vi "CreatEventsListFireRequestvi.vi"(10 "error in (no error)":errorcluster) -> (2 "error out":errorcluster, 3 "EvnLstFireRqst":T1 caption="EventsListFireRequest")   [LabVIEW 2020, in "CameraTestingProxy.lvlib" / "CameraTestingENI.lvclass"]
uses:
  CameraTestingENI.lvclass
  CameraTestingENI.lvclass/CameraTestingENI.ctl
  Community/TypeDef/RequestEventList.ctl
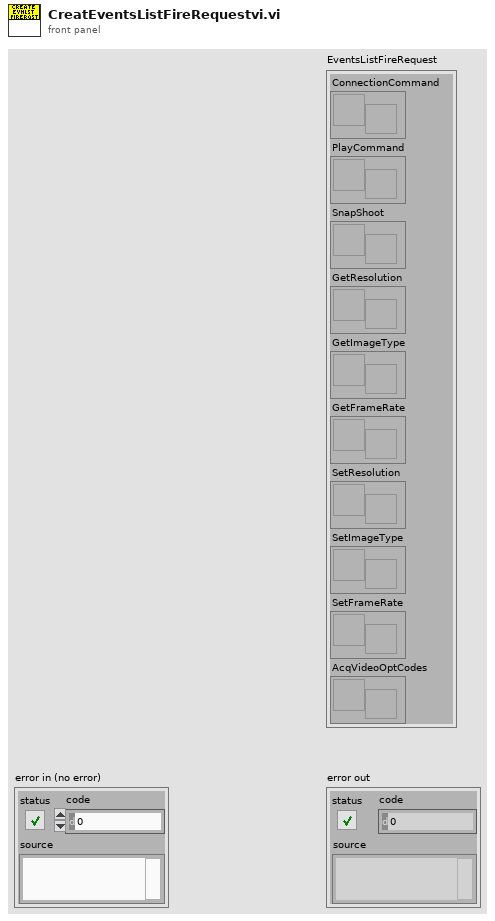
[diagram p1: front panel]
types:
  T1 = typedef "CameraTestingProxy.lvlib/CameraTestingENI.lvclass/RequestEventList.ctl" = cluster{"ConnectCmd":refnum<user-event>, "PlayCmd":refnum<user-event>, "SnapShoot":refnum<user-event>, "GetResolution":refnum<user-event>, "GetImageType":refnum<user-event>, "GetFrameRate":refnum<user-event>, "SetResolution":refnum<user-event>, "SetImageType":refnum<user-event>, "SetFrameRate":refnum<user-event>, "AcqVideoOptCodes":refnum<user-event>}
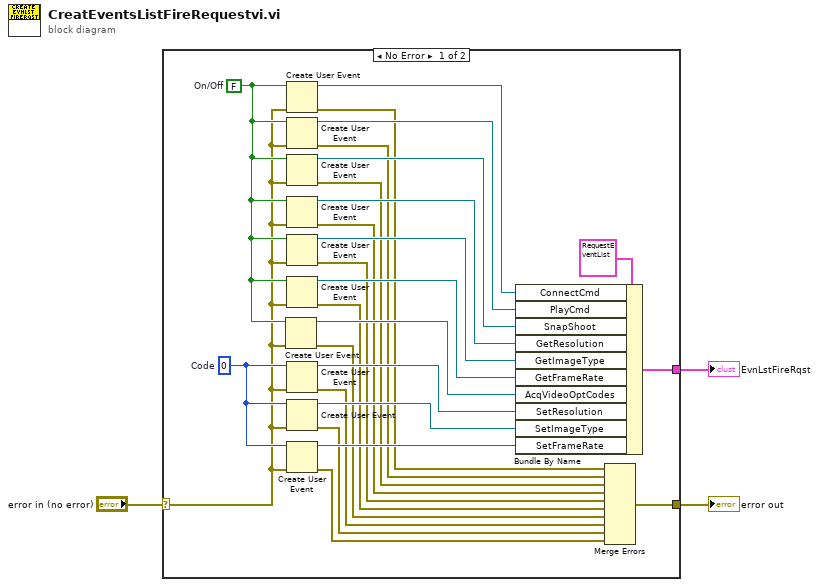
[diagram p0: block diagram]
diagram:
  n1 = case shown="No Error" "error in (no error)" {
    selector: "error in (no error)" -> [w15 w30]
    tunnel: [w16 _] -> w3
    tunnel: [w4 w30] -> w1
    frame No Error {
      w17 = u8 0  # Code
      w19 = FALSE  # On/Off
      n2 = Create User Event(user event datatype=w19, error in=w15) -> (user event=w18:refnum<user-event>, error out=w8:errorcluster)
      n3 = Create User Event(user event datatype=w19, error in=w15) -> (user event=w29:refnum<user-event>, error out=w14:errorcluster)
      n4 = Create User Event(user event datatype=w19, error in=w15) -> (user event=w28:refnum<user-event>, error out=w13:errorcluster)
      n5 = Create User Event(user event datatype=w19, error in=w15) -> (user event=w27:refnum<user-event>, error out=w12:errorcluster)
      n6 = Create User Event(user event datatype=w19, error in=w15) -> (user event=w26:refnum<user-event>, error out=w11:errorcluster)
      n7 = Create User Event(user event datatype=w19, error in=w15) -> (user event=w25:refnum<user-event>, error out=w10:errorcluster)
      n8 = Create User Event(user event datatype=w19, error in=w15) -> (user event=w24:refnum<user-event>, error out=w9:errorcluster)
      n9 = Create User Event(user event datatype=w17, error in=w15) -> (user event=w23:refnum<user-event>, error out=w7:errorcluster)
      n10 = Create User Event(user event datatype=w17, error in=w15) -> (user event=w22:refnum<user-event>, error out=w6:errorcluster)
      n11 = Create User Event(user event datatype=w17, error in=w15) -> (user event=w21:refnum<user-event>, error out=w5:errorcluster)
      n12 = Bundle By Name(cluster=T1 {"ConnectCmd"=refnum, "PlayCmd"=refnum, "SnapShoot"=refnum, "GetResolution"=refnum, "GetImageType"=refnum, "GetFrameRate"=refnum, "SetResolution"=refnum, "SetImageType"=refnum, "SetFrameRate"=refnum, "AcqVideoOptCodes"=refnum} ("EvnLstFireRqst"), "ConnectCmd"=w29, "PlayCmd"=w28, "SnapShoot"=w27, "GetResolution"=w26, "GetImageType"=w25, "GetFrameRate"=w24, "AcqVideoOptCodes"=w18, "SetResolution"=w23, "SetImageType"=w22, "SetFrameRate"=w21) -> (w16:T1)
      n13 = Merge Errors(w14, w13, w12, w11, w10, w9, w8, w7, w6, w5) -> (w4:errorcluster)
    }
    frame Error {
    }
  }
  "EvnLstFireRqst" <- w3
  "error out" <- w1
